vi "CLC_Gen3_L1_GUI.vi"() -> ()   [LabVIEW 2023, in "Clover_Cell.lvlib"]
uses:
  Clover_Cell.lvlib
panel:
  out "error out":errorcluster
  in  "Ethernet Setting":T1={"address"="192.168.100.111", "remote port or service name"=5025, "timeout ms (60000)"=10000}
  out "Status":bool
  in  "Ch2?":bool
  in  "Ch3?":bool
  in  "Ch4?":bool
  in  "Ch1?":bool
  in  "Ch3_phase":i32=32 min=0 max=63 step=1
  in  "Ch2_phase":i32=32 min=0 max=63 step=1
  in  "Ch1_phase":i32 min=0 max=63 step=1
  in  "Ch4_phase":i32 min=0 max=63 step=1
  in  "Ch4_gain":i32 min=0 max=15 step=1
  in  "Ch3_gain":i32 min=0 max=15 step=1
  in  "Ch2_gain":i32 min=0 max=15 step=1
  in  "Ch1_gain":i32 min=0 max=15 step=1
  in  "Polarity":u16(ring) items=["H", "V"]
  in  "TRXmode":u16(ring)=1 items=["Rx"=2, "Tx"=1]
  # "CLC_Gen3_L1 Setting GUI"
  # "Ch_On/OFF"
  # "Phase"
  # "Gain"
  # "Ch-1."
  # "Ch-2."
  # "Ch-3."
  # "Ch-4."
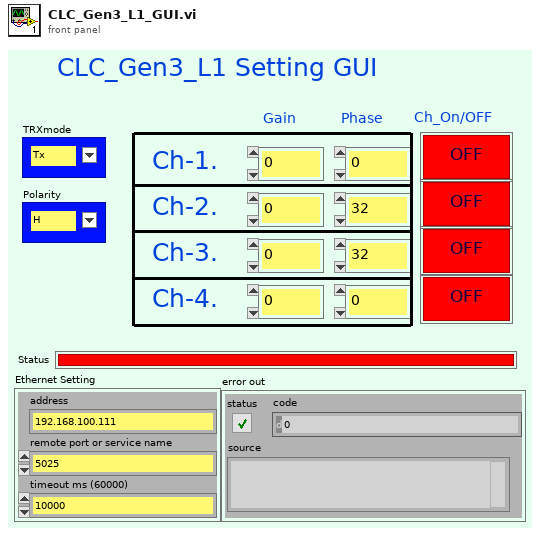
[diagram p1: front panel]
types:
  T1 = cluster{"address":string, "remote port or service name":u16, "timeout ms (60000)":i32}
  T2 = cluster{"Mode":u16, "Polarity":u16, "CH_ON/OFF":u16, "Channel":i32, "Gain":i32, "Phase":i32}
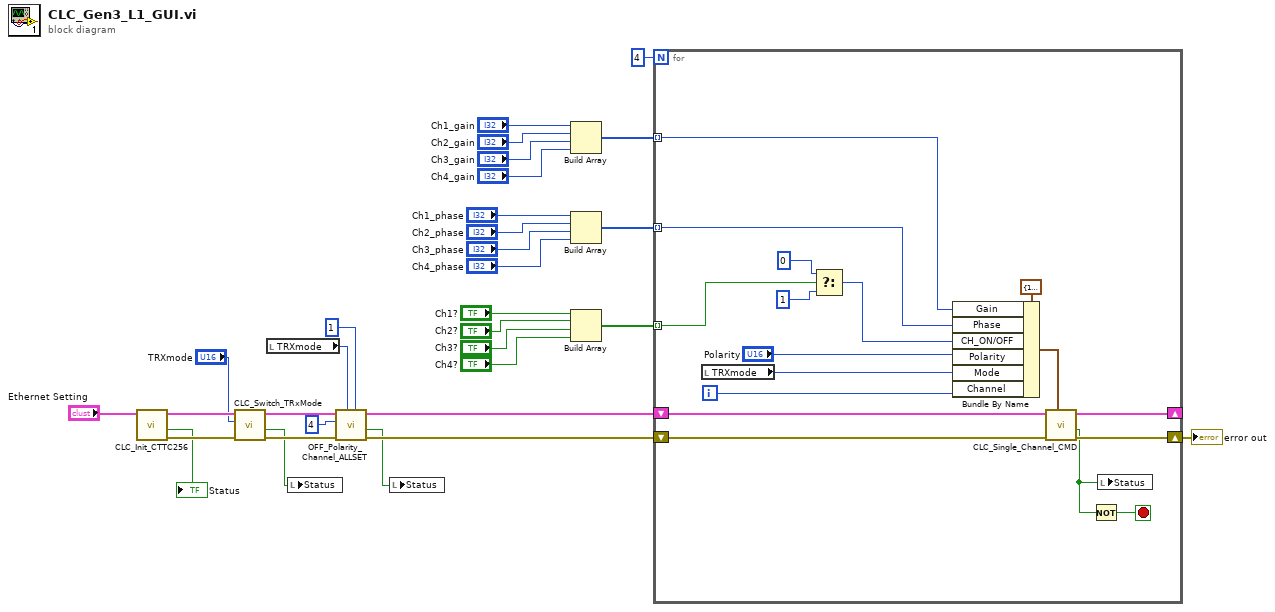
[diagram p0: block diagram]
diagram:
  n1 = call "CLC_Init_CTTC256.vi"("TCPIPin"="Ethernet Setting") -> ("error out"=w31:errorcluster, "Status"=→"Status":bool, "TCPIPin 2"=w28:T1)  [unwired: 8 in]
  n2 = call "CLC_Switch_TRxMode.vi"("error in (no error)"=w31, "Text Ring"="TRXmode", "TCPIPin"=w28) -> ("error out"=w30:errorcluster, "OK?"=w7:bool, "TCPIPin 2"=w25:T1)  [unwired: 6 in]
  n3 = local read "TRXmode"() -> (w24:u16)
  n4 = local write "Status"(w7) -> ()
  n5 = call "OFF_Polarity_Channel_ALLSET.vi"("CH_ON:0/OFF:1"=u16 1, "Mode"=w24, "error in"=w30, "Channel"=4, "TCPIPin"=w25) -> ("error out"=w10:errorcluster, "OK?"=w6:bool, "TCPIPout"=w9:T1)  [unwired: 4 in]
  n6 = local write "Status"(w6) -> ()
  n7 = Build Array("Ch1_gain", "Ch2_gain", "Ch3_gain", "Ch4_gain") -> (w5:i32[])
  n8 = Build Array("Ch1_phase", "Ch2_phase", "Ch3_phase", "Ch4_phase") -> (w4:i32[])
  n9 = Build Array("Ch1?", "Ch2?", "Ch3?", "Ch4?") -> (w3:bool[])
  n10 = for {
    N: 4 -> [_]
    shift-right: [w44] -> w1
    shift-left: w10 -> [w45]
    shift-right: [w43] -> _
    shift-left: w9 -> [w46]
    tunnel: w5 -> [w42] mode=indexing
    tunnel: w4 -> [w41] mode=indexing
    tunnel: w3 -> [w37] mode=indexing
    i -> [w40]
    stop <- w32 stop-if-true
    n11 = local read "TRXmode"() -> (w39:u16)
    n12 = Select(t=u16 0 ("CH_ON/OFF"), s=w37, f=u16 1 ("CH_ON/OFF")) -> (s? t:f=w34:u16)
    n13 = Bundle By Name(cluster=T2 {"Mode"=1, "Polarity"=1, "CH_ON/OFF"=1, "Channel"=0, "Gain"=0, "Phase"=0} ("Channel params"), "Gain"=w42, "Phase"=w41, "CH_ON/OFF"=w34, "Polarity"="Polarity", "Mode"=w39, "Channel"=w40) -> (w47:T2)
    n14 = call "CLC_Single_Channel_CMD.vi"("Channel params"=w47, "error in"=w45, "TCPIPin"=w46) -> ("error out"=w44:errorcluster, "OK?"=w33:bool, "TCPIPout"=w43:T1)  [unwired: 6 in]
    n15 = Not(x=w33) -> (.not. x?=w32:bool)
    n16 = local write "Status"(w33) -> ()
  }
  "error out" <- w1
